vi "QC Draw.vi"(1 "steering":T1={"control"={"rudder"=0, "aileron"=0}, "rotate"={"pitch"=3.9968028886505635e-15, "roll"=25.71428571428572, "yaw"=-69.79591836734694}, "pos"={"x"=0.0, "y"=0.0, "z"=-138.77551020408163}} {"control"."rudder" scale=-30.0..30.0; "control"."aileron" scale=-30.0..30.0; "rotate"."pitch" scale=-180.0..180.0; "rotate"."roll" scale=-180.0..180.0; "rotate"."yaw" scale=-180.0..180.0; "pos"."x" scale=-10.0..10.0; "pos"."y" scale=-20.0..20.0; "pos"."z" scale=-200.0..200.0}, 2 "Picture Reference":refnum<vi>) -> (0 "picture out 2":picture)   [LabVIEW 2011]
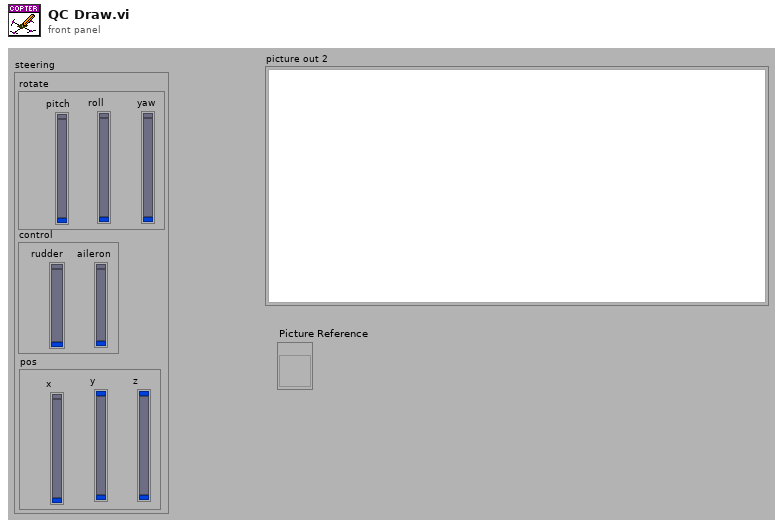
[diagram p1: front panel]
types:
  T1 = cluster{"control":cluster{"rudder":i32, "aileron":i32}, "rotate":cluster{"pitch":dbl, "roll":dbl, "yaw":dbl}, "pos":cluster{"x":dbl, "y":dbl, "z":dbl}}
  T2 = typedef "LVBoundsTypeDef.ctl" = cluster{"Width":u32, "Height":u32}
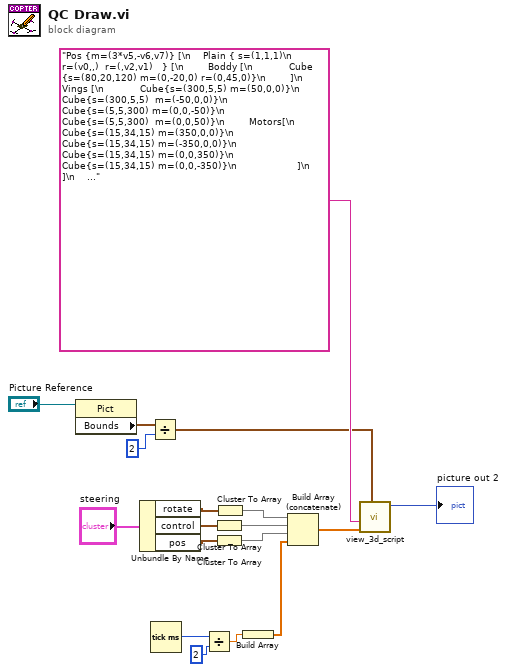
[diagram p0: block diagram]
diagram:
  n1 = property class="Pict"(reference="Picture Reference") -> ("Bounds"=w4:T2)  [unwired: 1 in, 2 out]
  n2 = Unbundle By Name("steering") -> ("rotate"=w5:cluster{"pitch":dbl, "roll":dbl, "yaw":dbl}, "control"=w6:cluster{"rudder":i32, "aileron":i32}, "pos"=w7:cluster{"x":dbl, "y":dbl, "z":dbl})
  n3 = Divide(x=w4, y=2) -> (x/y=w2:cluster{"Width":dbl, "Height":dbl})
  n4 = Tick Count (ms)() -> (millisecond timer value=w13:u32)
  n5 = Divide(x=w13, y=u16 2) -> (x/y=w12:dbl)
  n6 = Cluster To Array(cluster=w6) -> (array=w17:i32[])
  n7 = Cluster To Array(cluster=w7) -> (array=w16:dbl[])
  n8 = Cluster To Array(cluster=w5) -> (array=w18:dbl[])
  n9 = Build Array(w12) -> (w15:dbl[])
  n10 = Build Array (concatenate)(w18, w17, w16, w15) -> (w11:dbl[])
  n11 = call "view_3d_script.vi"("center"=w2, "variables"=w11, "script"="Pos {m=(3*v5,-v6,v7)} [\n    Plain { s=(1,1,1)\n                   r=(v0,,)  r=(,v2,v1)   } [\n        Boddy [\n            Cube {s=(80,20,120) m=(0,-20,0) r=(0,45,0)}\n        ]\n        Vings [\n            Cube{s=(300,5,5) m=(50,0,0)}\n            Cube{s=(300,5,5)  m=(-50,0,0)}\n            Cube{s=(5,5,300) m=(0,0,-50)}\n            Cube{s=(5,5,300)  m=(0,0,50)}\n        Motors[\n                Cube{s=(15,34,15) m=(350,0,0)}\n                Cube{s=(15,34,15) m=(-350,0,0)}\n                Cube{s=(15,34,15) m=(0,0,350)}\n                Cube{s=(15,34,15) m=(0,0,-350)}\n                    ]\n        ]\n    ]\n]") -> ("picture out"=→"picture out 2":picture)  [unwired: 3 in, 2 out]
